vi "Main Action Process Ctrl_NameArr.vi"(7 "Action":T1(ring)=enum."Delete & Check", 8 "error in":errorcluster, 9 "index":i32, 10 "Add Action Que":string[](array[string])) -> (0 "Finish":bool, 1 "Delete Action":string, 2 "Count":i32, 3 "Read Action":string, 4 "error out":errorcluster)   [LabVIEW 2019]
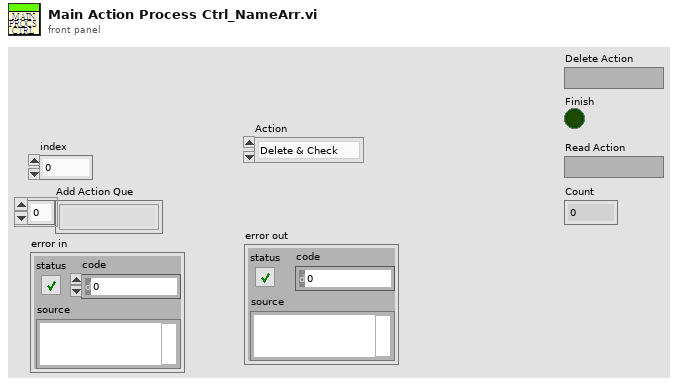
[diagram p1: front panel]
types:
  T1 = enum16{"Initial", "Add", "Read", "Delete & Check"}
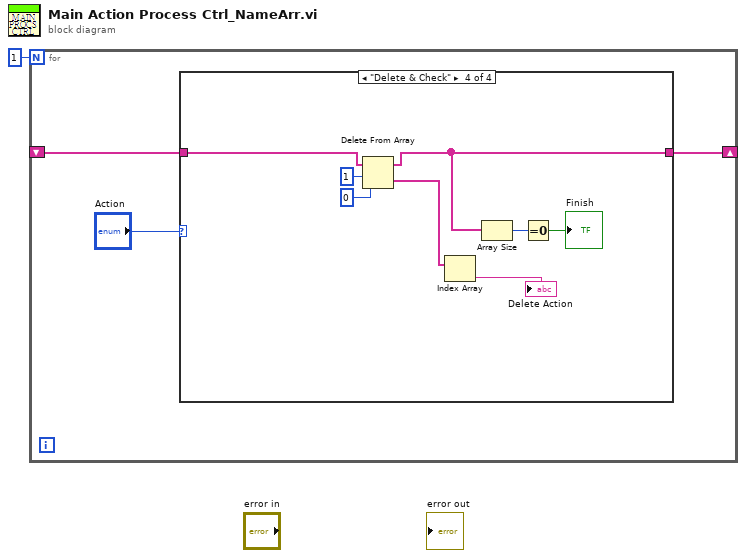
[diagram p0: block diagram]
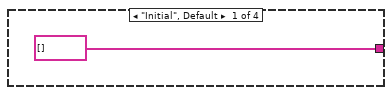
[diagram p2: hidden frame]
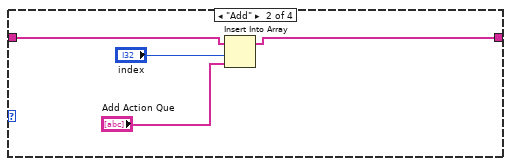
[diagram p3: hidden frame]
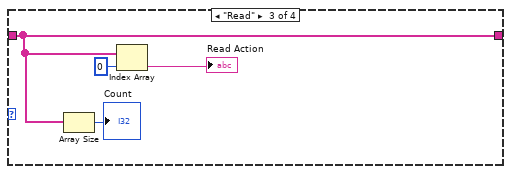
[diagram p4: hidden frame]
diagram:
  n1 = for {
    N: 1 -> [_]
    shift-right: [w4] -> _
    shift-left: _ -> [w3]
    n2 = case shown="\"Delete & Check\"" "Action" {
      tunnel: [string[] [] w8 w11 w20] -> w4
      tunnel: w3 -> [_ w9 w11 w21]
      frame "Initial", Default {
      }
      frame "Add" {
        n3 = Insert Into Array(array=w9, index="index", new element="Add Action Que") -> (w8:string[])
      }
      frame "Read" {
        n4 = Array Size(array=w11) -> (size(s)=→"Count":i32)
        n5 = Index Array(array=w11, index=0) -> (element=→"Read Action":string)
      }
      frame "Delete & Check" {
        n6 = Delete From Array(array=w21, length=1, index=0) -> (deleted portion=w17:string[], array with subset deleted=w20:string[])
        n7 = Index Array(array=w17) -> (element=→"Delete Action":string)  [unwired: 1 in]
        n8 = Array Size(array=w20) -> (size(s)=w15:i32)
        n9 = Equal To 0?(x=w15) -> (x = 0?=→"Finish":bool)
      }
    }
  }
